vi "2D boolean array show.vi"(0 "Input array":bool[][](array[boolean])=[[FALSE]] caption="Auto Focus Success", 1 "Caption.Text":string="Auto Focus Success", 2 "Columns":u8 min=1, 3 "Rows":u8 min=1, 4 "Colors [4]":cluster{u32, u32}[](array[cluster]), 5 "Auto close (s)":u32=15) -> ()   [LabVIEW 2018]
panel:
  out "Windows close (s)":u32 caption="Window closes in"
  in  "Done":bool
  # "s"
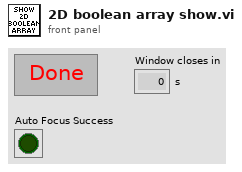
[diagram p1: front panel]
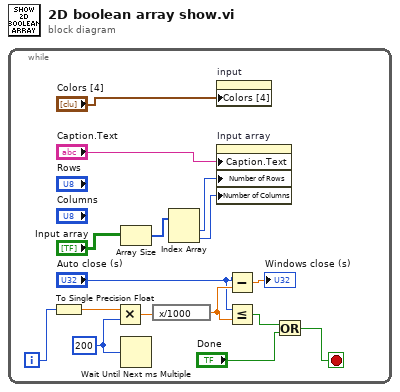
[diagram p0: block diagram]
diagram:
  n1 = while {
    i -> [w9]
    stop <- w7 stop-if-true
    w10 = u32 200 ("millisecond multiple")
    n2 = To Single Precision Float(number=w9) -> (single precision float=w1:sgl)
    n3 = Multiply(x=w1, y=w10) -> (x*y=w2:sgl)
    n4 = Array Size(array="Input array") -> (size(s)=w14:i32[])
    n5 = Wait Until Next ms Multiple(millisecond multiple=w10) -> ()  [unwired: 1 out]
    n6 = expression code="x/1000"(w2) -> (w5:sgl)
    n7 = Index Array(array=w14) -> (element #1=w13:i32, element #2=w12:i32)  [unwired: 2 in]
    n8 = property on="input" class="Bool (strict)"("Colors [4]"="Colors [4]") -> ()  [unwired: 2 in, 2 out]
    n9 = property on="Input array" class="Arr (strict)"("Caption.Text"="Caption.Text", "Number of Rows"=w13, "Number of Columns"=w12) -> ()  [unwired: 2 in, 2 out]
    n10 = Subtract(x="Auto close (s)", y=w5) -> (x-y=→"Windows close (s)":sgl)
    n11 = Less Or Equal?(x="Auto close (s)", y=w5) -> (x <= y?=w4:bool)
    n12 = Or(x=w4, y="Done") -> (x .or. y?=w7:bool)
  }
